vi "Actor Core.vi"(8 "error in":cluster{"状态":bool, "代码":i32, "源":string} caption="错误输入", 11 "冷却器UI":refnum<class "Live User Controller.lvclass">) -> (0 "error out":cluster{"状态":bool, "代码":i32, "源":string} caption="错误输出", 3 "操作者输出":refnum<class "Actor.lvclass">)   [LabVIEW 2013, in "Live User Controller.lvclass"]
doc: "Actor Core.vi包含操作者的主要消息处理循环。操作者通常位于该循环中，在各种消息到达时对消息进行处理。如Do.vi消息返回任何错误，该循环将停止运行，错误代码43将被作为“无错误停止”的标准信号发送给调用方。如需更改上述行为，可在子孙类的Handle Error.vi中对该部分逻辑进行重写。"
uses:
  Live User Controller.lvclass
  <vilib>/ActorFramework/Actor/Actor.lvclass
  <vilib>/ActorFramework/Actor/Actor.lvclass/Actor.ctl
  Cooler Controller/Cooler Controller/Cooler Controller.lvclass/Cooler Controller.ctl
  <vilib>/ActorFramework/Message Enqueuer/Message Enqueuer.lvclass/Message Enqueuer.ctl
  Evaporative Cooler Controller/Evaporative Cooler Controller/Evaporative Cooler Controller.lvclass
  Air Cooler Application/Load Into Sub Panel Msg/Load Into Sub Panel Msg.lvclass/Load Into Sub Panel Msg.ctl
  Cooler Controller/Change Desired Temperature Msg/Change Desired Temperature Msg.lvclass/Change Desired Temperature Msg.ctl
  <vilib>/ActorFramework/Stop Msg/Stop Msg.lvclass/Stop Msg.ctl
  <vilib>/ActorFramework/Message Enqueuer/Init from Existing Queue.vi
  <vilib>/ActorFramework/Message Enqueuer/Enqueue.vi
  <vilib>/ActorFramework/Message Enqueuer/Enqueue Critical.vi
  <vilib>/ActorFramework/Message Priority Queue/Priority Enqueue.vi
  <vilib>/ActorFramework/Message Enqueuer/Message Enqueuer.lvclass
  Air Cooler Application/Load Into Sub Panel Msg/Load Into Sub Panel Msg.lvclass
  Cooler Controller/Change Desired Temperature Msg/Change Desired Temperature Msg.lvclass
  <vilib>/ActorFramework/Stop Msg/Stop Msg.lvclass
  Cooler Controller/Cooler Controller/Cooler Controller.lvclass
panel:
  in  "停止":bool
  out "水泵处于活动状态？":dbl(slide) scale=0.0..25.0
  out "检测到故障":bool
  in  "待维持的温度":dbl=75.0
  out "实际温度":dbl(slide) scale=60.0..120.0
  out "检测到故障":bool
  out "风扇B":bool
  out "风扇A":bool
  out "水槽":dbl(slide)=10.459183673469388 scale=0.0..25.0
  out "泵状态":bool
  # "水泵启动后风扇加速5秒钟。"
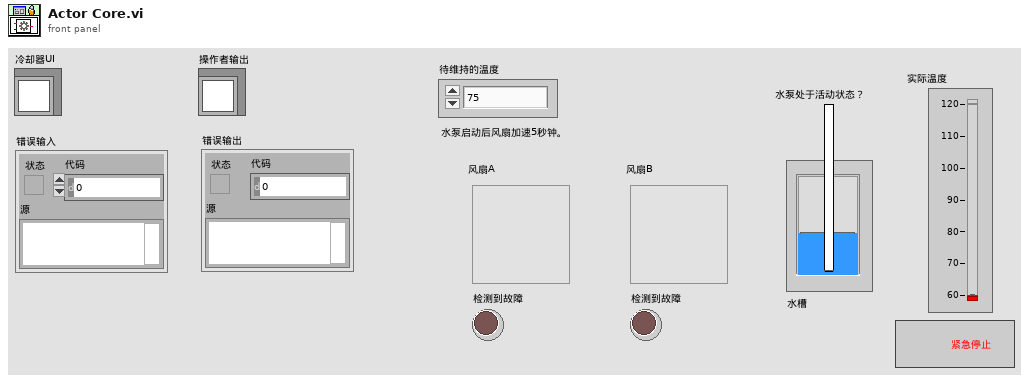
[diagram p1: front panel]
types:
  T1 = cluster{"Pump Status":bool, "Pump Level":dbl, "Pump Dir":bool}
  T2 = cluster{"实际温度":refnum<vi>, "风扇A":refnum<vi>, "检测到故障":refnum<vi>, "风扇B":refnum<vi>, "检测到故障":refnum<vi>, "泵状态":refnum<vi>, "水槽":refnum<vi>}
  T3 = enum32{"Invalid", "Standard", "Closed", "Hidden", "Minimized", "Maximized"}
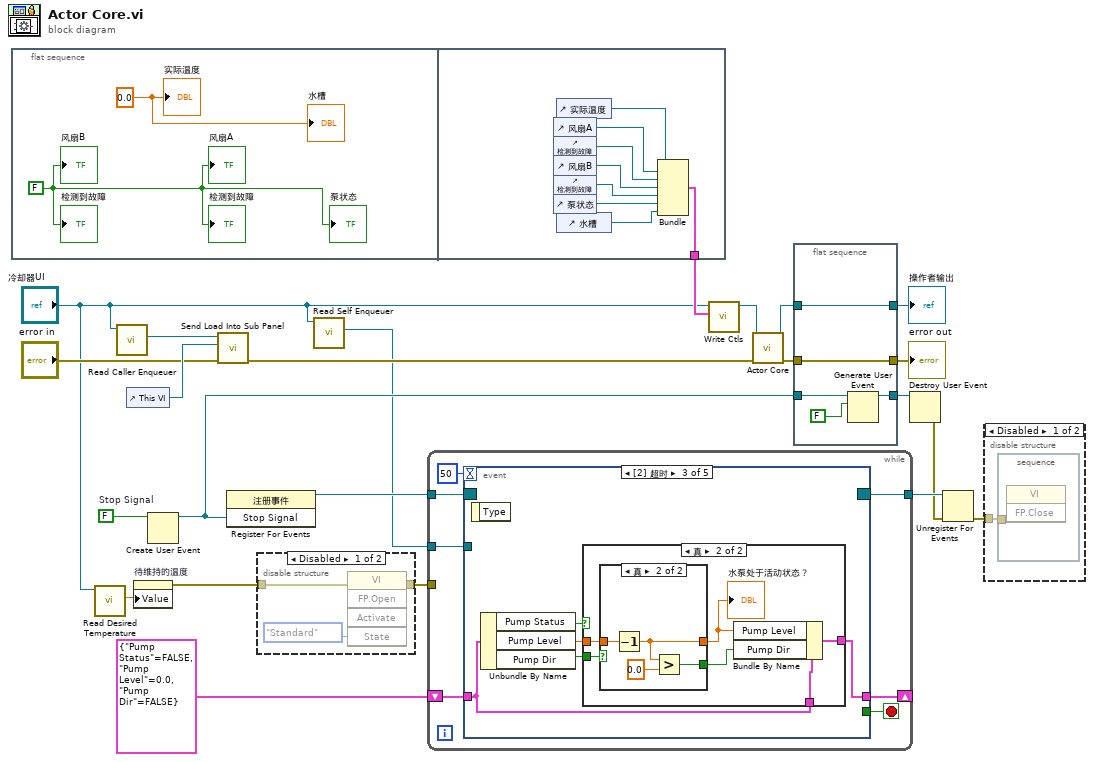
[diagram p0: block diagram]
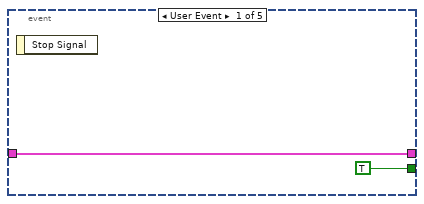
[diagram p4: hidden frame]
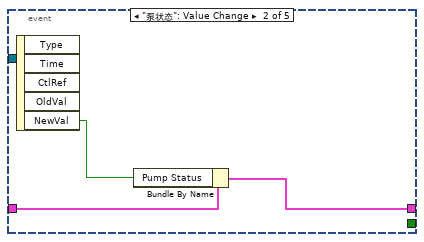
[diagram p5: hidden frame]
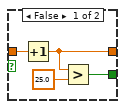
[diagram p7: hidden frame]
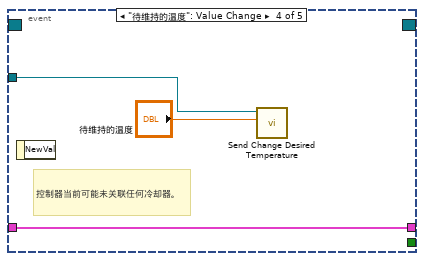
[diagram p8: hidden frame]
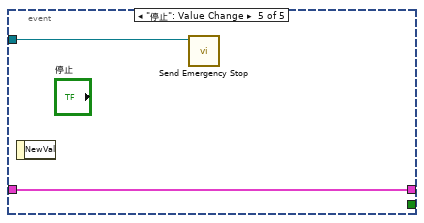
[diagram p9: hidden frame]
diagram:
  w20 = FALSE  # Stop Signal
  n1 = flat-sequence {
    tunnel: [w28] -> w22
    frame #0 {
      w24 = 0.0 ("value")
      w25 = FALSE
      "实际温度" <- w24
      "风扇A" <- w25
      "风扇B" <- w25
      "检测到故障" <- w25
      "检测到故障" <- w25
      "泵状态" <- w25
      "水槽" <- w24
    }
    frame #1 {
      n2 = control-ref of="风扇A"() -> (w30:refnum<vi>)
      n3 = control-ref of="检测到故障"() -> (w31:refnum<vi>)
      n4 = control-ref of="风扇B"() -> (w29:refnum<vi>)
      n5 = control-ref of="检测到故障"() -> (w32:refnum<vi>)
      n6 = control-ref of="泵状态"() -> (w27:refnum<vi>)
      n7 = control-ref of="实际温度"() -> (w33:refnum<vi>)
      n8 = control-ref of="水槽"() -> (w26:refnum<vi>)
      n9 = Bundle("实际温度"=w33, "风扇A"=w30, "检测到故障"=w31, "风扇B"=w29, "检测到故障"=w32, "泵状态"=w27, "水槽"=w26) -> (w28:T2)  [unwired: 1 in]
    }
  }
  n10 = call "Read Desired Temperature.vi"("冷却器的控制器输入"="冷却器UI") -> ("待维持的温度"=w7:dbl)  [unwired: 10 in]
  n11 = call <vilib>:"Read Caller Enqueuer.vi"("Actor"="冷却器UI") -> ("Caller Enqueuer"=w6:refnum<class "Message Enqueuer.lvclass">)  [unwired: 10 in]
  n12 = control-ref of="This VI"() -> (w5:refnum<vi>)
  n13 = property on="待维持的温度" class="DigNum (严格)"("Value"=w7) -> (error out=w8:errorcluster)  [unwired: 2 in, 1 out]
  n14 = Create User Event(user event datatype=w20) -> (user event=w16:refnum<user-event>)  [unwired: 1 in, 1 out]
  n15 = call "Send Load Into Sub Panel.vi"("error in (no error)"="error in", "用于子面板的VI"=w5, "消息待入队列"=w6) -> ("error out"=w3:cluster{"状态":bool, "代码":i32, "源":string})  [unwired: 8 in]
  n16 = register-events(w16) -> (reference out=w21:refnum<event-registration>)  [unwired: 2 in, 1 out]
  n17 = disable-structure shown="Disabled" {
    disable-tunnel: [w35 _] -> w10
    disable-tunnel: w8 -> [w34 _]
    frame Disabled {
      n18 = invoke class="VI" method="FP.Open"(error in=w34, "State"=T3."Standard") -> (error out=w35:errorcluster)  [unwired: 3 in, 4 out]
    }
    frame Enabled {
    }
  }
  n19 = call <vilib>:"Read Self Enqueuer.vi"("Actor"="冷却器UI") -> ("Self Enqueuer"=w1:refnum<class "Message Enqueuer.lvclass">)  [unwired: 10 in]
  n20 = while {
    tunnel: w21 -> [w43]
    tunnel: [w42] -> w19
    shift-right: [w40] -> _
    shift-left: T1 {"Pump Status"=FALSE, "Pump Level"=0.0, "Pump Dir"=FALSE} -> [w39]
    tunnel: w10 -> [_]
    tunnel: w1 -> [w37]
    stop <- w41 stop-if-true
    n21 = event shown="[2] 超时" {
      selector: w43 -> [_ _ _ _ _]
      dyn-events: [_ _ _ _ _] -> w42
      timeout: 50 -> [_ _ _ _ _]
      tunnel: [TRUE _ _ _ _] -> w41
      tunnel: [w44 w47 w51 w71 w73] -> w40
      tunnel: w39 -> [w44 w48 w50 w71 w73]
      tunnel: w37 -> [_ _ _ w70 w72]
      event User Event {
        n22 = event-data() -> ()  [unwired: 1 in, 1 out]
      }
      event "泵状态": Value Change {
        n23 = event-data() -> ("NewVal"=w46:bool)  [unwired: 1 in, 4 out]
        n24 = Bundle By Name(cluster=w48, "Pump Status"=w46) -> (w47:T1)
      }
      event Timeout {
        n25 = event-data() -> ()  [unwired: 1 in, 1 out]
        n26 = Unbundle By Name(w50) -> ("Pump Status"=w53:bool, "Pump Level"=w49:dbl, "Pump Dir"=w52:bool)
        n27 = case shown="真" w53 {
          tunnel: w52 -> [_ w60]
          tunnel: [w54 w59] -> w51
          tunnel: w50 -> [w54 w58]
          tunnel: w49 -> [_ w57]
          frame False {
          }
          frame True {
            n28 = case shown="真" w60 {
              tunnel: w57 -> [w64 w68]
              tunnel: [w63 w67] -> w55
              tunnel: [w61 w65] -> w56
              frame False {
                n29 = Increment(x=w64) -> (x+1=w63:dbl)
                n30 = Greater?(x=w63, y=25.0) -> (0:w61:bool)
              }
              frame True {
                n31 = Decrement(x=w68) -> (x-1=w67:dbl)
                n32 = Greater?(x=w67, y=0.0) -> (0:w65:bool)
              }
            }
            "水泵处于活动状态？" <- w55
            n33 = Bundle By Name(cluster=w58, "Pump Level"=w55, "Pump Dir"=w56) -> (w59:T1)
          }
        }
      }
      event "待维持的温度": Value Change {
        # "控制器当前可能未关联任何冷却器。"
        n34 = event-data() -> ()  [unwired: 1 in, 1 out]
        n35 = call "Send Change Desired Temperature.vi"("待维持的温度"="待维持的温度", "消息待入队列"=w70) -> ()  [unwired: 9 in, 1 out]
      }
      event "停止": Value Change {
        n36 = event-data() -> ()  [unwired: 1 in, 1 out]
        n37 = call <vilib>:"Send Emergency Stop.vi"("Message Enqueuer"=w72) -> ()  [unwired: 10 in, 1 out]
      }
    }
  }
  n38 = call "Write Ctls.vi"("控件"=w22, "冷却器UI输入"="冷却器UI") -> ("冷却器UI输出"=w23:refnum<class "Live User Controller.lvclass">)  [unwired: 9 in]
  n39 = call-parent "Actor Core.vi"("error in"=w3, "Actor in"=w23) -> ("error out"=w12:errorcluster, "Actor out"=w14:refnum<class "Actor.lvclass">)  [unwired: 8 in]
  n40 = flat-sequence {
    tunnel: [w78] -> w17
    tunnel: w16 -> [w77]
    tunnel: w14 -> [w76]
    tunnel: [w76] -> w15
    tunnel: w12 -> [w75]
    tunnel: [w75] -> w13
    frame #0 {
      n41 = Generate User Event(user event=w77, event data cluster=FALSE ("Stop Signal")) -> (user event out=w78:refnum<user-event>)  [unwired: 2 in, 1 out]
    }
  }
  n42 = Destroy User Event(user event=w17) -> (error out=w18:errorcluster)  [unwired: 1 in]
  n43 = Unregister For Events(event registration refnum=w19, error in=w18) -> (error out=w9:errorcluster)
  n44 = disable-structure shown="Disabled" {
    disable-tunnel: w9 -> [w79 _]
    frame Disabled {
      n45 = stacked-sequence {
        tunnel: w79 -> [_]
        frame #0 {
          n46 = invoke class="VI" method="FP.Close"() -> ()  [unwired: 3 in, 3 out]
        }
      }
    }
    frame Enabled {
    }
  }
  "error out" <- w13
  "操作者输出" <- w15
